vi "Write Rates.vi"(8 "error in (no error)":errorcluster, 10 "Rates":dbl[](array[numeric]), 11 "Temperature Controller Driver in":refnum<class "Temperature Controller Driver.lvclass">) -> (0 "error out":errorcluster, 3 "Temperature Controller Driver out":refnum<class "Temperature Controller Driver.lvclass">)   [LabVIEW 2024, in "Temperature Controller Driver.lvclass"]
uses:
  Temperature Controller Driver.lvclass
  Temperature Controller Driver.lvclass/Temperature Controller Driver.ctl
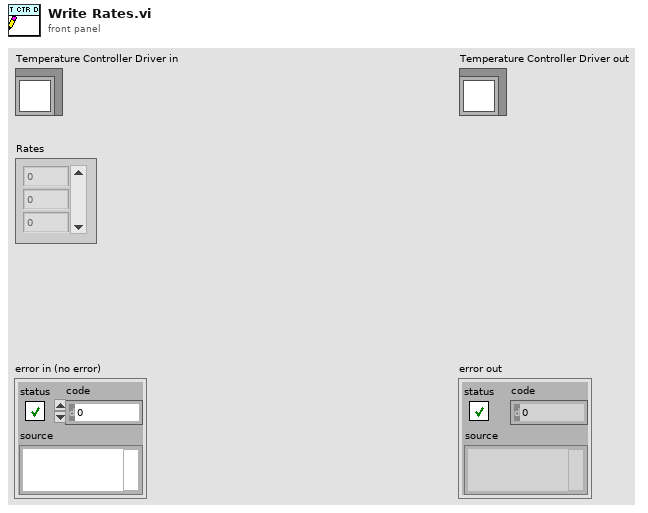
[diagram p1: front panel]
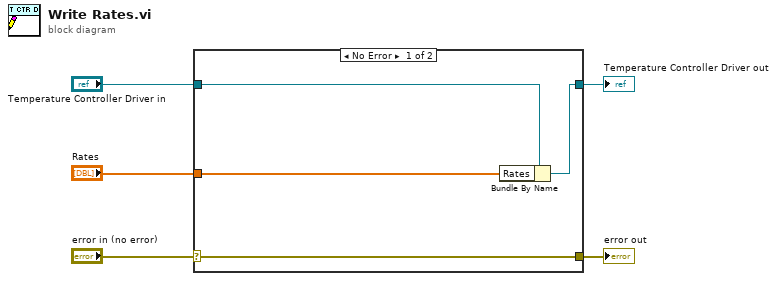
[diagram p0: block diagram]
diagram:
  n1 = case shown="No Error" "error in (no error)" {
    selector: "error in (no error)" -> [w9 w10]
    tunnel: [w9 w10] -> w4
    tunnel: [w7 w11] -> w2
    tunnel: "Temperature Controller Driver in" -> [w8 w11]
    tunnel: "Rates" -> [w6 _]
    frame No Error {
      n2 = Bundle By Name(cluster=w8, "Rates"=w6) -> (w7:refnum<class "Temperature Controller Driver.lvclass">)
    }
    frame Error {
    }
  }
  "error out" <- w4
  "Temperature Controller Driver out" <- w2
